vi "FTW-ProjectItemManager-Enumerate.vi"(0 "Project Item Manager":refnum<class "FTW-ProjectItemManager.lvclass">, 5 "Tag Regex Filter (blank returns all tags)":string, 11 "error in":errorcluster) -> (4 "Project Item Manager out":refnum<class "FTW-ProjectItemManager.lvclass">, 6 "Matching Tags":string[](array[string]), 8 "Regex Results":cluster{"Match":string, "Submatches":string[]}[](array[cluster]), 15 "error out":errorcluster)   [LabVIEW 2012, in "FTW-ProjectItemManager.lvclass"]
uses:
  FTW-ProjectItemManager.lvclass
  FTW-ProjectItemManager.lvclass/FTW-ProjectItemManager.ctl
panel:
  # "Inputs"
  # "Outputs"
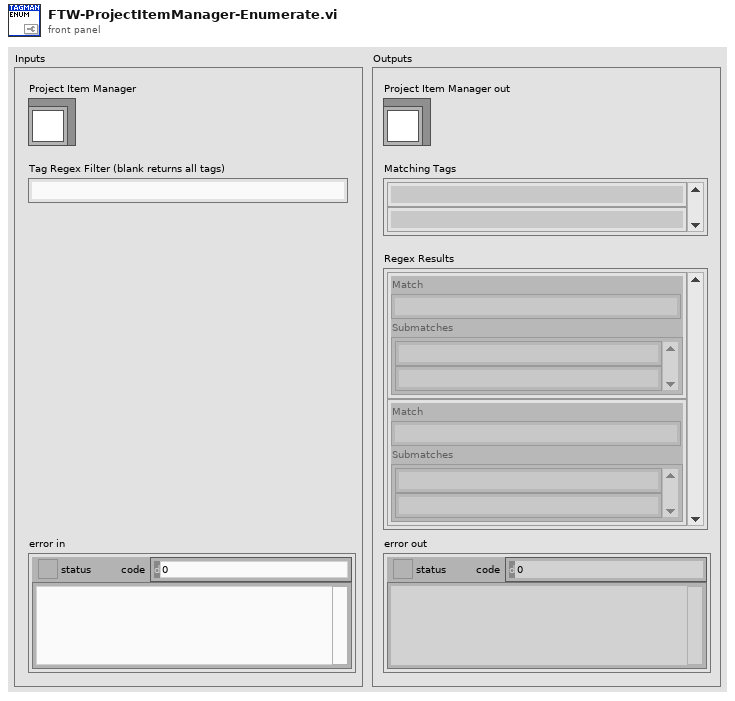
[diagram p1: front panel]
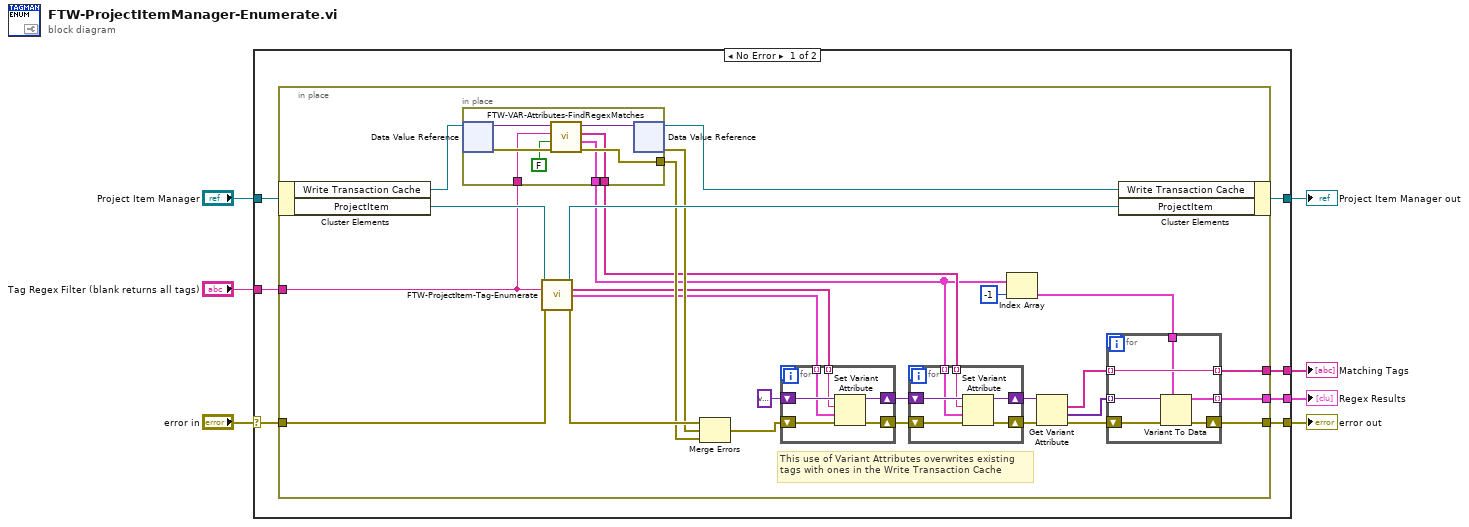
[diagram p0: block diagram]
diagram:
  n1 = case shown="No Error" "error in" {
    selector: "error in" -> [w14 w69]
    tunnel: [w13 w69] -> w7
    tunnel: [w8 w68] -> w5
    tunnel: "Project Item Manager" -> [w9 w68]
    tunnel: "Tag Regex Filter (blank returns all tags)" -> [w12 _]
    tunnel: [w11 _] -> w2
    tunnel: [w10 _] -> w1
    frame No Error {
      n2 = in-place {
        in-place-border: w14 -> [w41]
        in-place-border: [w22] -> w13
        in-place-border: w12 -> [w33]
        in-place-border: [w20] -> w11
        in-place-border: [w16] -> w10
        # "This use of Variant Attributes overwrites existing\ntags with ones in the Write Transaction Cache"
        n3 = in-place-cluster #1(w9) -> ("Write Transaction Cache"=w38:refnum<data-value>, "ProjectItem"=w40:refnum<vi>)
        n4 = in-place {
          in-place-border: [w63] -> w34
          in-place-border: w33 -> [w62]
          in-place-border: [w61] -> w27
          in-place-border: [w60] -> w19
          n5 = in-place-dvr #2(w38) -> (w67:variant, w65:errorcluster)
          n6 = call "FTW-VAR-Attributes-FindRegexMatches.vi"("error in"=w65, "Force Literal Match?"=FALSE, "Regex Match for Attributes"=w62, "Variant"=w67) -> ("error out"=w63:errorcluster, "Regex Results"=w60:cluster{"Match":string, "Submatches":string[]}[], "Matching Attributes"=w61:string[], "Variant out"=w66:variant)  [unwired: 4 in]
          n7 = in-place-dvr #2(w66) -> (w37:refnum<data-value>, w35:errorcluster)
        }
        n8 = call "FTW-ProjectItem-Tag-Enumerate.vi"("ProjectItem"=w40, "Tag Name Regex Filter (blank returns all tags)"=w33, "error in"=w41) -> ("ProjectItem out"=w39:refnum<vi>, "Matching Tags"=w30:string[], "Regex Results"=w15:cluster{"Match":string, "Submatches":string[]}[], "error out"=w36:errorcluster)  [unwired: 9 in]
        n9 = Merge Errors(w36, w35, w34) -> (w31:errorcluster)
        n10 = for {
          shift-right: [w58] -> w29
          shift-left: variant -> [w59]
          shift-right: [w56] -> w28
          shift-left: w31 -> [w57]
          tunnel: w30 -> [w55] mode=indexing
          tunnel: w15 -> [w54] mode=indexing
          n11 = Set Variant Attribute(Variant=w59, name=w55, value=w54, error in=w57) -> (Variant out=w58:variant, error out=w56:errorcluster)  [unwired: 1 out]
        }
        n12 = for {
          shift-right: [w52] -> w25
          shift-left: w29 -> [w53]
          shift-right: [w50] -> w26
          shift-left: w28 -> [w51]
          tunnel: w27 -> [w49] mode=indexing
          tunnel: w19 -> [w48] mode=indexing
          n13 = Set Variant Attribute(Variant=w53, name=w49, value=w48, error in=w51) -> (Variant out=w52:variant, error out=w50:errorcluster)  [unwired: 1 out]
        }
        n14 = Index Array(array=w19, index=-1) -> (element=w17:cluster{"Match":string, "Submatches":string[]})
        n15 = Get Variant Attribute(Variant=w25, error in=w26) -> (names=w21:string[], values=w24:variant[], error out=w23:errorcluster)  [unwired: 2 in, 1 out]
        n16 = for {
          shift-right: [w46] -> w22
          shift-left: w23 -> [w47]
          tunnel: w21 -> [w45] mode=indexing
          tunnel: [w45] -> w20 mode=indexing
          tunnel: w17 -> [w43]
          tunnel: w24 -> [w44] mode=indexing
          tunnel: [w42] -> w16 mode=indexing
          n17 = Variant To Data(error in=w47, type=w43, Variant=w44) -> (data=w42:cluster{"Match":string, "Submatches":string[]}, error out=w46:errorcluster)
        }
        n18 = in-place-cluster #1("Write Transaction Cache"=w37, "ProjectItem"=w39) -> (w8:refnum<class "FTW-ProjectItemManager.lvclass">)
      }
    }
    frame Error {
    }
  }
  "error out" <- w7
  "Project Item Manager out" <- w5
  "Matching Tags" <- w2
  "Regex Results" <- w1
